vi "IP array list.vi"(11 "IP STATUS(in)":T1) -> (3 "IP STATUS(out)":T1)   [LabVIEW 2011]
uses:
  UDP packet capture/ArrayIpAddressesAndReportingCheckbox.ctl
panel:
  in  "IP STATUS(set)":T1
  in  "Cancel Button":bool
  in  "OK Button":bool
  # "IP Addresses and Reporting"
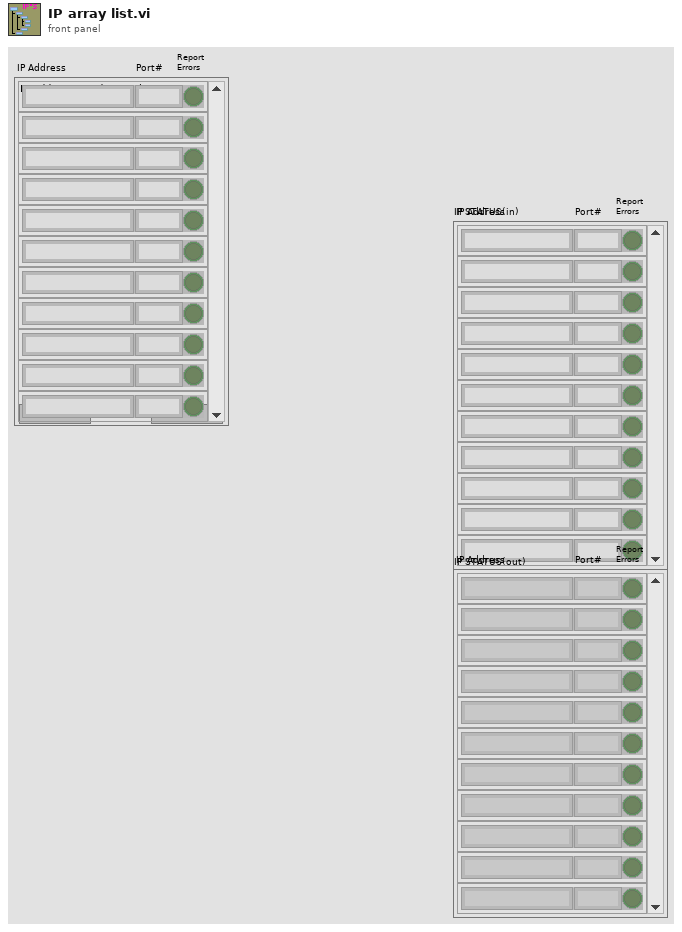
[diagram p1: front panel]
types:
  T1 = typedef "ArrayIpAddressesAndReportingCheckbox.ctl" = cluster{"IpAddress":string, "Report Errors":bool, "IpAddress 2":string}[]
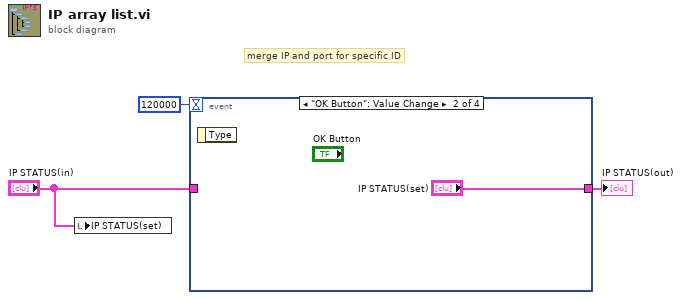
[diagram p0: block diagram]
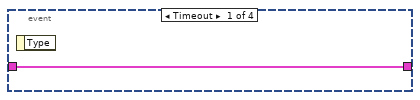
[diagram p2: hidden frame]
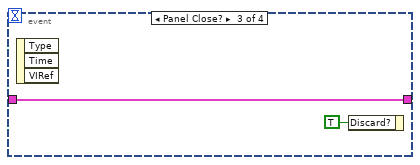
[diagram p3: hidden frame]
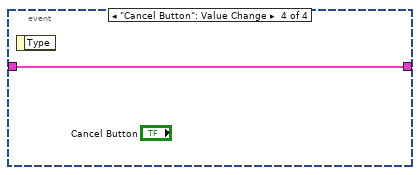
[diagram p4: hidden frame]
diagram:
  # "merge IP and port for specific ID"
  n1 = local write "IP STATUS(set)"("IP STATUS(in)") -> ()
  n2 = event shown="[1] \"OK Button\": Value Change" {
    selector: _ -> [_ _ _ _]
    dyn-events: _ -> [_ _ _ _]
    timeout: 120000 -> [_ _ _ _]
    tunnel: "IP STATUS(in)" -> [w4 _ w7 w8]
    tunnel: [w4 "IP STATUS(set)" w7 w8] -> w2
    event Timeout {
      n3 = event-data() -> ()  [unwired: 1 in, 1 out]
    }
    event "OK Button": Value Change {
      n4 = event-data() -> ()  [unwired: 1 in, 1 out]
    }
    event Panel Close? {
      n5 = event-data() -> ()  [unwired: 1 in, 3 out]
      n6 = event-data("Discard?"=TRUE) -> ()  [unwired: 1 in, 1 out]
    }
    event "Cancel Button": Value Change {
      n7 = event-data() -> ()  [unwired: 1 in, 1 out]
    }
  }
  "IP STATUS(out)" <- w2
